vi "Move_VXM_Win7.vi"(1 "error in (no error)":errorcluster, 2 "Single Axis Movement (mm)":dbl, 3 "Motor Speed (mm/sec)":dbl, 4 "Motor Number":i32=1 min=1 max=3 step=1) -> (0 "error out":errorcluster)   [LabVIEW 2017]
panel:
  out "Port Chars 2":string
  out "Port Chars":string
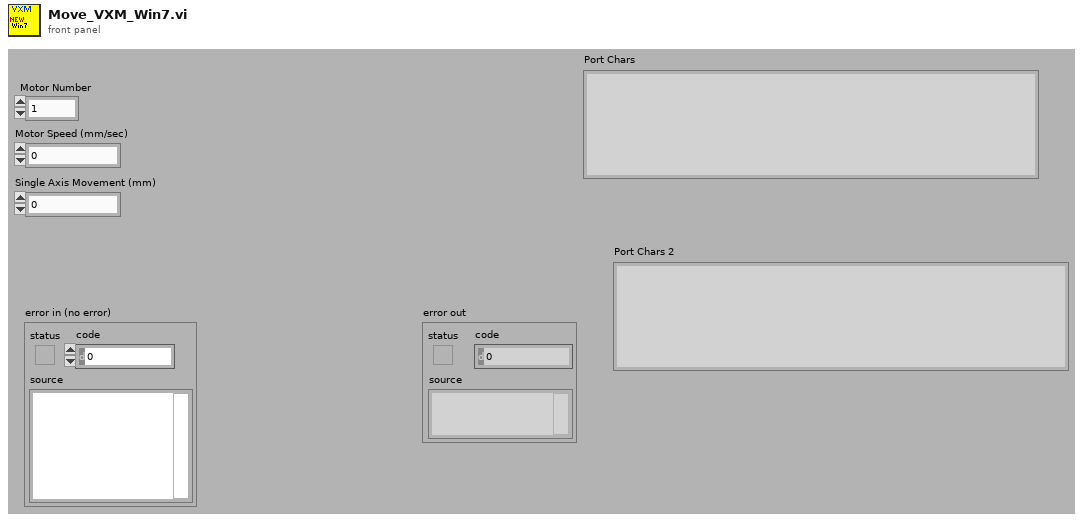
[diagram p1: front panel]
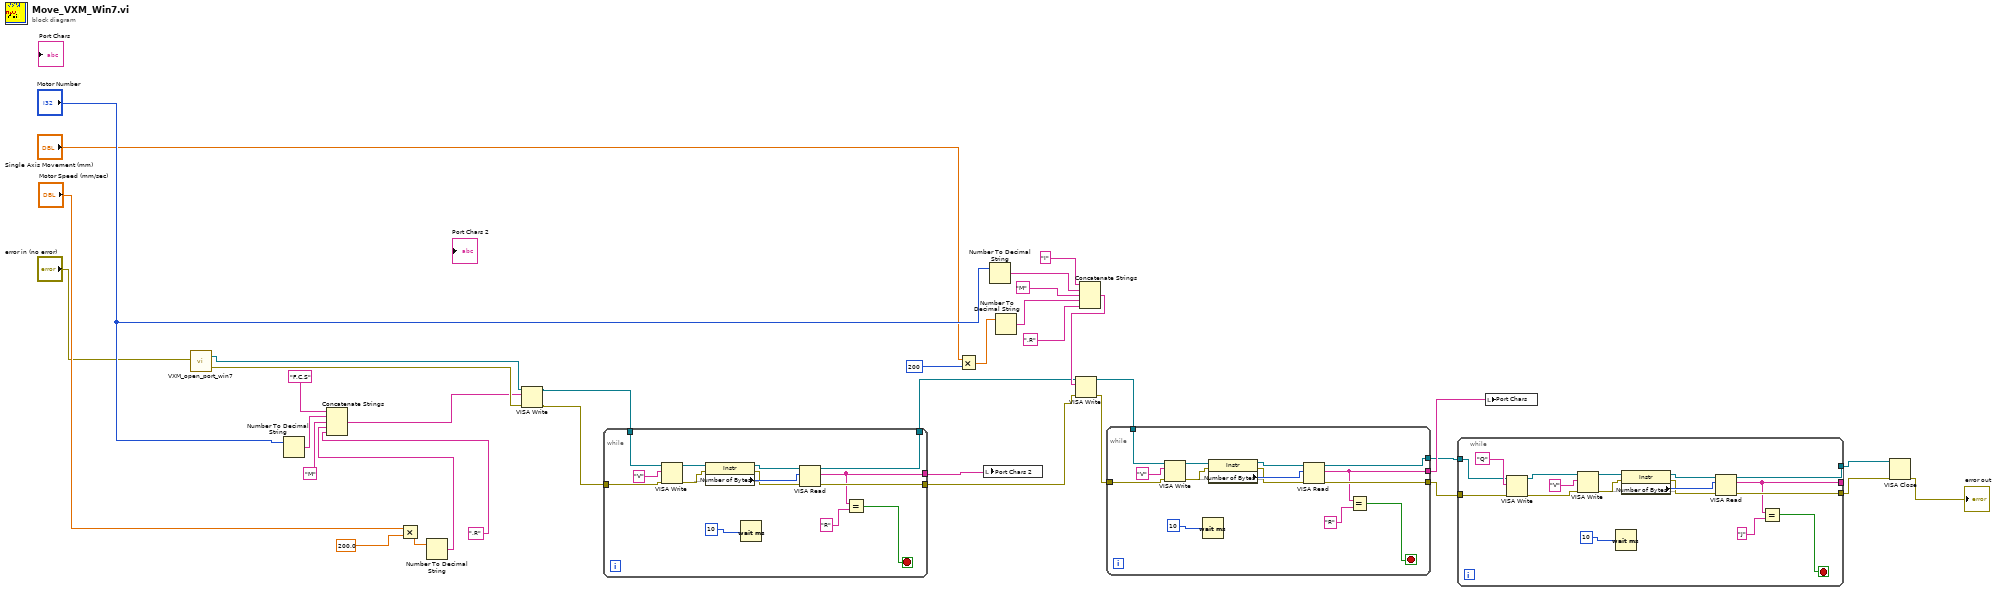
[diagram p0: block diagram]
diagram:
  n1 = call "VXM_open_port_win7.vi"("error in (no error)"="error in (no error)") -> ("VISA resource name out"=w15:refnum<visa-resource-name>, "error out"=w17:errorcluster)
  n2 = Number To Decimal String(number="Motor Number") -> (decimal integer string=w34:string)  [unwired: 1 in]
  n3 = Multiply(x="Motor Speed (mm/sec)", y=200.0) -> (x*y=w32:dbl)
  n4 = Number To Decimal String(number=w32) -> (decimal integer string=w30:string)  [unwired: 1 in]
  n5 = Concatenate Strings("F,C,S", w34, "M", w30, ",R") -> (w16:string)
  n6 = VISA Write(VISA resource name=w15, write buffer=w16, error in (no error)=w17) -> (VISA resource name out=w12:refnum<visa-resource-name>, error out=w11:errorcluster)  [unwired: 1 out]
  n7 = while {
    tunnel: w11 -> [w46]
    tunnel: w12 -> [w45]
    tunnel: [w38] -> w10
    tunnel: [w41] -> w9
    tunnel: [w40] -> w8
    stop <- w37 stop-if-true
    n8 = VISA Write(VISA resource name=w45, write buffer="V", error in (no error)=w46) -> (VISA resource name out=w48:refnum<visa-resource-name>, error out=w47:errorcluster)  [unwired: 1 out]
    n9 = property class="Instr"(reference=w48, error in=w47) -> (reference out=w43:refnum<visa-resource-name>, error out=w42:errorcluster, "Serial Settings:Number of Bytes at Serial Port"=w44:u32)
    n10 = Wait (ms)(milliseconds to wait=10) -> ()  [unwired: 1 out]
    n11 = VISA Read(VISA resource name=w43, byte count=w44, error in (no error)=w42) -> (VISA resource name out=w41:refnum<visa-resource-name>, read buffer=w38:string, error out=w40:errorcluster)  [unwired: 1 out]
    n12 = Equal?(x=w38, y="R") -> (x = y?=w37:bool)
  }
  n13 = Multiply(x="Single Axis Movement (mm)", y=200) -> (x*y=w27:dbl)
  n14 = local write "Port Chars 2"(w10) -> ()
  n15 = Number To Decimal String(number="Motor Number") -> (decimal integer string=w24:string)  [unwired: 1 in]
  n16 = Number To Decimal String(number=w27) -> (decimal integer string=w22:string)  [unwired: 1 in]
  n17 = Concatenate Strings("I", w24, "M", w22, ",R") -> (w14:string)
  n18 = VISA Write(VISA resource name=w9, write buffer=w14, error in (no error)=w8) -> (VISA resource name out=w7:refnum<visa-resource-name>, error out=w6:errorcluster)  [unwired: 1 out]
  n19 = while {
    tunnel: w6 -> [w60]
    tunnel: w7 -> [w59]
    tunnel: [w53] -> w5
    tunnel: [w55] -> w1
    tunnel: [w50] -> w2
    stop <- w52 stop-if-true
    n20 = VISA Write(VISA resource name=w59, write buffer="V", error in (no error)=w60) -> (VISA resource name out=w62:refnum<visa-resource-name>, error out=w61:errorcluster)  [unwired: 1 out]
    n21 = Wait (ms)(milliseconds to wait=10) -> ()  [unwired: 1 out]
    n22 = property class="Instr"(reference=w62, error in=w61) -> (reference out=w57:refnum<visa-resource-name>, error out=w56:errorcluster, "Serial Settings:Number of Bytes at Serial Port"=w58:u32)
    n23 = VISA Read(VISA resource name=w57, byte count=w58, error in (no error)=w56) -> (VISA resource name out=w50:refnum<visa-resource-name>, read buffer=w53:string, error out=w55:errorcluster)  [unwired: 1 out]
    n24 = Equal?(x=w53, y="R") -> (x = y?=w52:bool)
  }
  n25 = while {
    tunnel: [w71] -> _
    tunnel: [w74] -> w3
    tunnel: [w73] -> w4
    tunnel: w2 -> [w66]
    tunnel: w1 -> [w67]
    stop <- w70 stop-if-true
    n26 = VISA Write(VISA resource name=w66, write buffer="Q", error in (no error)=w67) -> (VISA resource name out=w65:refnum<visa-resource-name>, error out=w64:errorcluster)  [unwired: 1 out]
    n27 = VISA Write(VISA resource name=w65, write buffer="V", error in (no error)=w64) -> (VISA resource name out=w79:refnum<visa-resource-name>, error out=w78:errorcluster)  [unwired: 1 out]
    n28 = Wait (ms)(milliseconds to wait=10) -> ()  [unwired: 1 out]
    n29 = property class="Instr"(reference=w79, error in=w78) -> (reference out=w76:refnum<visa-resource-name>, error out=w75:errorcluster, "Serial Settings:Number of Bytes at Serial Port"=w77:u32)
    n30 = VISA Read(VISA resource name=w76, byte count=w77, error in (no error)=w75) -> (VISA resource name out=w74:refnum<visa-resource-name>, read buffer=w71:string, error out=w73:errorcluster)  [unwired: 1 out]
    n31 = Equal?(x=w71, y="J") -> (x = y?=w70:bool)
  }
  n32 = local write "Port Chars"(w5) -> ()
  n33 = VISA Close(VISA resource name=w3, error in (no error)=w4) -> (error out=→"error out":errorcluster)
